vi "Connect.vi"(8 "error in (no error)":errorcluster, 9 "timeout in ms (10000)":i32=10000, 11 "Communication in":refnum<class "IP_Communication.lvclass">) -> (0 "error out":errorcluster, 3 "Communication out":refnum<class "IP_Communication.lvclass">)   [LabVIEW 2020, in "Communication Classes.lvlib" / "IP_Communication.lvclass"]
uses:
  IP_Communication.lvclass
  IP_Communication.lvclass/IP_Communication.ctl
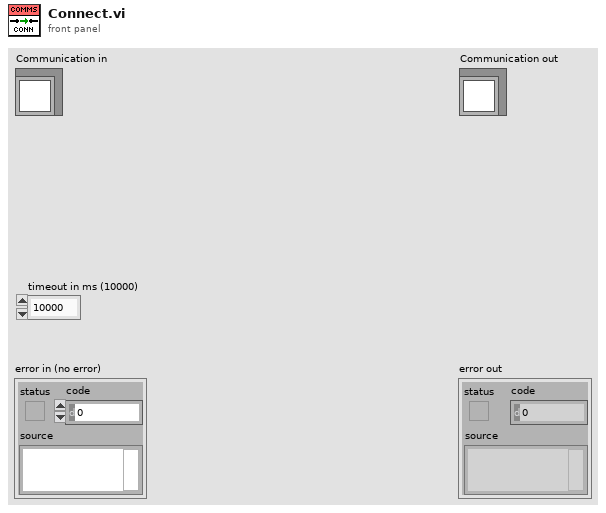
[diagram p1: front panel]
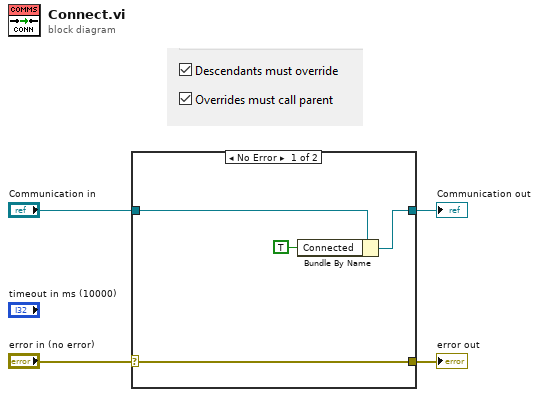
[diagram p0: block diagram]
diagram:
  n1 = case shown="No Error" "error in (no error)" {
    selector: "error in (no error)" -> [w8 w10]
    tunnel: [w8 w10] -> w3
    tunnel: [w5 w9] -> w1
    tunnel: "Communication in" -> [w7 w9]
    frame No Error {
      n2 = Bundle By Name(cluster=w7, "Connected"=TRUE) -> (w5:refnum<class "IP_Communication.lvclass">)
    }
    frame Error {
    }
  }
  "error out" <- w3
  "Communication out" <- w1
